vi "hdf5-repack-close.vi"(8 "error in":errorcluster, 11 "ref in":T1 format="%.0x") -> (0 "error out":errorcluster)   [LabVIEW 2016]
uses:
  <vilib>/addons/h5labview2/base/hid_t.ctl
  <vilib>/addons/h5labview2/file/H5Fmode.ctl
  <vilib>/addons/h5labview2/file/H5F.lvlib
  <vilib>/addons/h5labview2/attrib/H5A.lvlib
  <vilib>/addons/h5labview2/group/H5G.lvlib
panel:
  # "HDF5 datasets which are frequently extended occupy more disk space than necessary\nThis VI repacks the file and closes it"
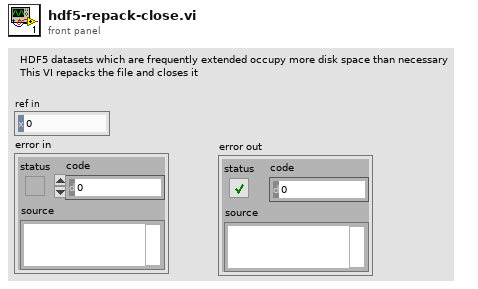
[diagram p1: front panel]
types:
  T1 = typedef "hid_t.ctl" = i32
  T2 = typedef "H5F.lvlib/H5Fmode.ctl" = enum16{"read-only", "read-write", "overwrite", "create new", "open or create"}
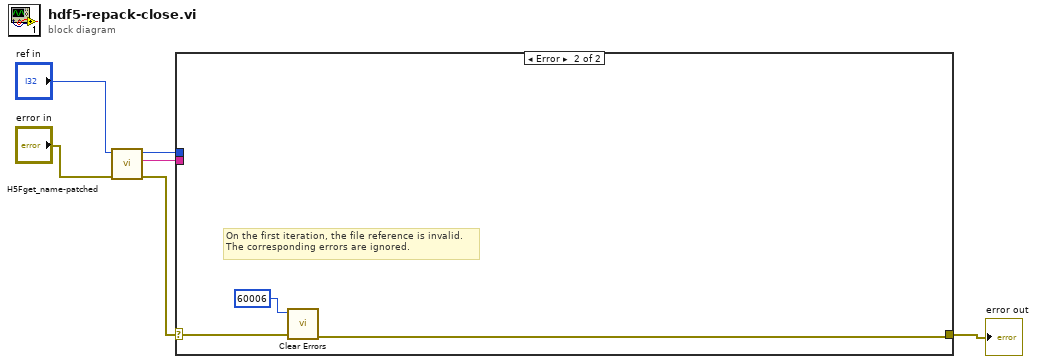
[diagram p0: block diagram]
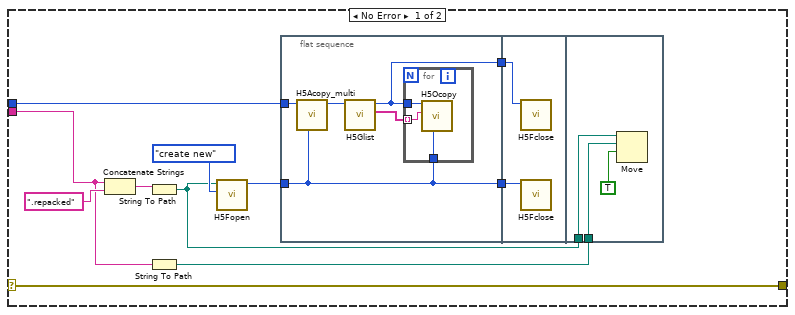
[diagram p2: hidden frame]
diagram:
  n1 = call "H5Fget_name-patched.vi"("error in (no error)"="error in", "ref in"="ref in") -> ("error out"=w4:errorcluster, "name"=w5:string, "ref out"=w6:T1)  [unwired: 7 in]
  n2 = case shown="Error" w4 {
    selector: w4 -> [w7 w33]
    tunnel: w6 -> [w16 _]
    tunnel: w5 -> [w9 _]
    tunnel: [w7 w32] -> w2
    frame No Error {
      n3 = Concatenate Strings(w9, ".repacked" ("string")) -> (w14:string)
      n4 = String To Path(string=w14) -> (path=w10:path)
      n5 = String To Path(string=w9) -> (path=w8:path)
      n6 = call <vilib>:"H5Fopen.vi"("mode (read-only)"=H5Fmode."create new", "path"=w10) -> ("ref out"=w13:T1)  [unwired: 8 in, 1 out]
      n7 = flat-sequence {
        tunnel: w16 -> [w20]
        tunnel: w13 -> [w18]
        tunnel: [w19] -> w12
        tunnel: [w18] -> w11
        tunnel: w12 -> [w27]
        tunnel: w11 -> [w26]
        tunnel: w10 -> [w29]
        tunnel: w8 -> [w28]
        frame #0 {
          n8 = call <vilib>:"H5Acopy_multi.vi"("dest in"=w18, "src in"=w20) -> ("src out"=w22:T1)  [unwired: 8 in, 1 out]
          n9 = call <vilib>:"H5Glist.vi"("ref in"=w22) -> ("names"=w21:string[], "ref out"=w19:T1)  [unwired: 7 in, 2 out]
          n10 = for {
            tunnel: w19 -> [w25]
            tunnel: w21 -> [w24] mode=indexing
            tunnel: w18 -> [w23]
            n11 = call <vilib>:"H5Ocopy.vi"("dest in"=w23, "src name (.)"=w24, "src in"=w25) -> ()  [unwired: 7 in, 2 out]
          }
        }
        frame #1 {
          n12 = call <vilib>:"H5Fclose.vi"("ref"=w27) -> ()  [unwired: 10 in, 1 out]
          n13 = call <vilib>:"H5Fclose.vi"("ref"=w26) -> ()  [unwired: 10 in, 1 out]
        }
        frame #2 {
          n14 = Move(source path=w29, 9:TRUE ("overwrite (F)"), 10:w28) -> ()  [unwired: 2 in, 3 out]
        }
      }
    }
    frame Error {
      # "On the first iteration, the file reference is invalid.\nThe corresponding errors are ignored."
      n15 = call <vilib>:"Clear Errors.vi"("error in (no error)"=w33, "specific error code to clear (0: all)"=60006) -> ("error out"=w32:errorcluster)  [unwired: 4 in, 1 out]
    }
  }
  "error out" <- w2
